vi "ME235ProjectVI.vi"() -> ()   [LabVIEW 2019]
uses:
  Serial - Settings.ctl
panel:
  out "XP2 Time":u8(graph)
  out "YP2 Time":u8(graph)
  out "YC1 Time":u8(graph)
  out "XC1 Time":u8(graph)
  in  "Speed Factor  Car 2":i32
  out "YC 1":u8[](array[numeric]) format="%x"
  out "XC1":u8[](array[numeric]) format="%x"
  out "YC2":u8[](array[numeric]) format="%x"
  out "XC2":u8[](array[numeric]) format="%x"
  in  "Set initial Y Car 2":dbl=1.3
  in  "Set initial X Car 2":dbl=2.6
  in  "?":bool
  in  "Time of Simulation in s":u8=5
  in  "command":u8=5
  out "XY Graph":cluster{u8[], u8[]}[](graph)
  out "Car Close By STOP":bool
  out "XY coordinates":u8[](array[numeric]) format="%x"
  out "return count":u32
  out "unsigned byte array":u8[](array[numeric])
  out "Packet Echo":u8[](array[numeric]) format="%x"
  out "read buffer":string
  in  "VISA resource name":refnum<visa-resource-name>="COM1"
  in  "Serial Settings":T1={"baud rate"=115200, "data bits"=8, "parity"=enum."None", "stop bits"=10, "flow control"=0} {"flow control" items=["None"=0, "XON/XOFF"=1, "RTS/CTS"=2, "DTR/DSR"=4]; "stop bits" items=["1.0"=10, "1.5"=15, "2.0"=20]; "data bits" min=5 max=8 step=1; "baud rate" items=["75"=75, "110"=110, "134"=134, "150"=150, "300"=300, "600"=600, "1200"=1200, "1800"=1800, "2400"=2400, "4800"=4800, "7200"=7200, "9600"=9600, "14400"=14400, "19200"=19200, "28800"=28800, "38400"=38400, "56000"=56000, "57600"=57600, "115200"=115200, "128000"=128000, "230400"=230400]}
  # "SIMULATION OF COLLISION DETECTION AND AVOIDANCE FOR 2 CARS"
  # "CAR 1 POSITION COMES FROM THE GPS INSIDE IT"
  # "CAR 1 INITIAL POS - X - 2, Y - 5, CAR 1 SPEED IS FACTOR 1"
  # "POSITIONS IN M, SPEED FACTOR"
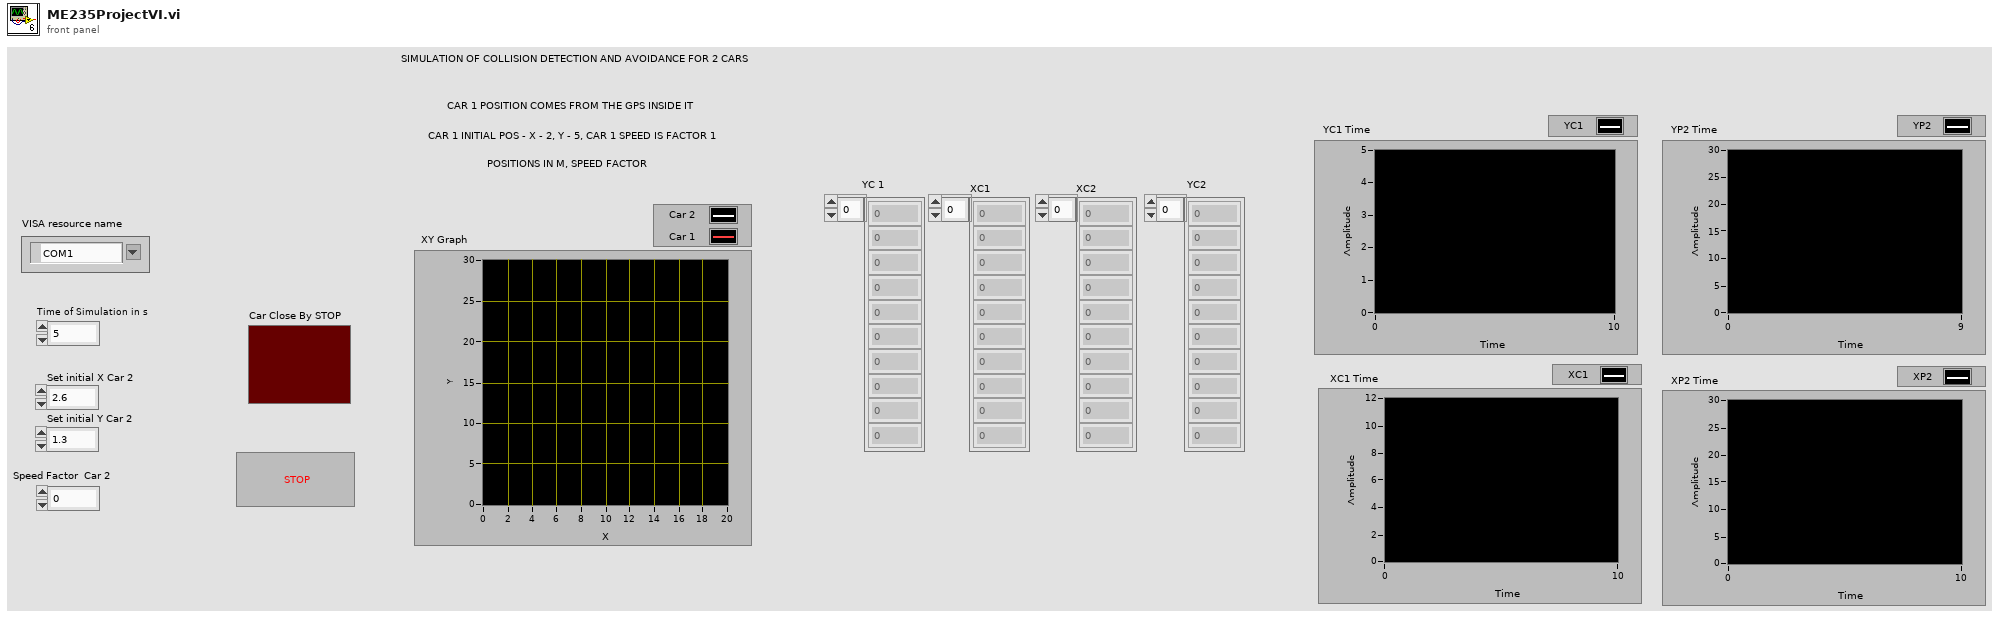
[diagram p1: front panel]
types:
  T1 = typedef "Serial - Settings.ctl" = cluster{"baud rate":u32, "data bits":u16, "parity":enum16{"None", "Odd", "Even", "Mark", "Space"}, "stop bits":u16, "flow control":u16}
  T2 = cluster{"Packet_Size":u8, "command":u8, "buffer":u8[]}
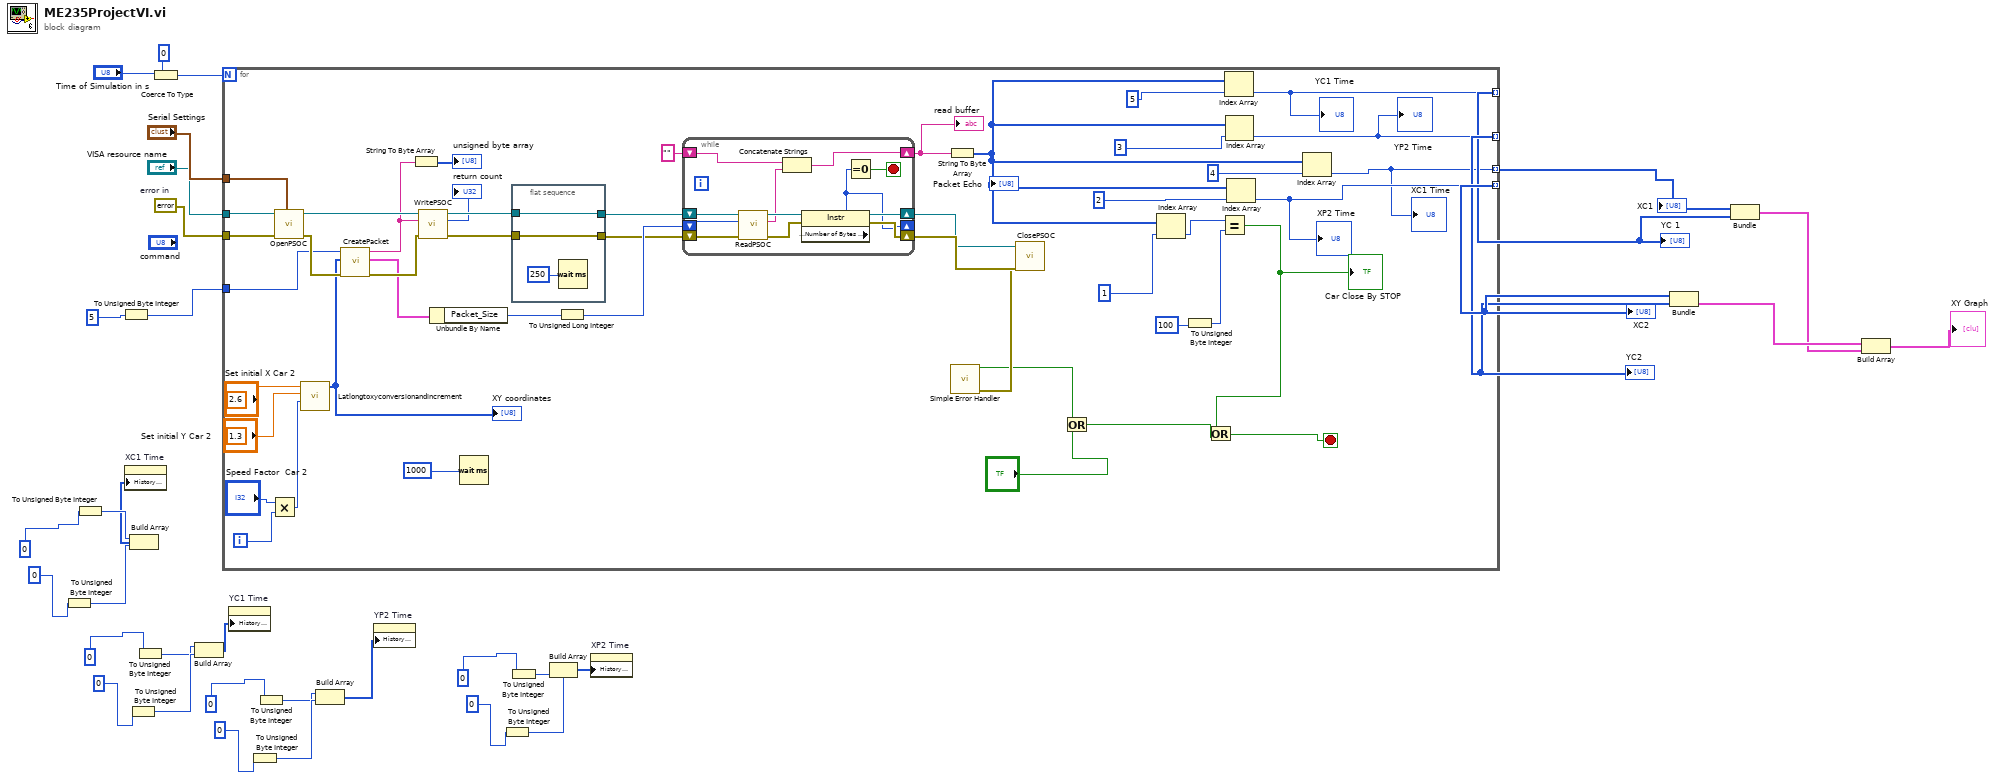
[diagram p0: block diagram]
diagram:
  w33 = errorcluster {"status"=FALSE, "code"=0, "source"=""}  # error in
  n1 = To Unsigned Byte Integer(number=0) -> (unsigned 8bit integer=w18:u8)
  n2 = To Unsigned Byte Integer(number=0) -> (unsigned 8bit integer=w17:u8)
  n3 = To Unsigned Byte Integer(number=5) -> (unsigned 8bit integer=w21:u8)
  n4 = To Unsigned Byte Integer(number=0) -> (unsigned 8bit integer=w13:u8)
  n5 = Build Array(w17, w18) -> (w16:u8[])
  n6 = property on="XC1 Time" class="WFChart (strict)"("History Data"=w16) -> ()  [unwired: 2 in, 2 out]
  n7 = To Unsigned Byte Integer(number=0) -> (unsigned 8bit integer=w12:u8)
  n8 = Coerce To Type(0:"Time of Simulation in s", 1:0) -> (2:w26:i32)
  n9 = Build Array(w12, w13) -> (w11:u8[])
  n10 = for {
    N: w26 -> [_]
    tunnel: "Serial Settings" -> [w82]
    tunnel: "VISA resource name" -> [w81]
    tunnel: w33 -> [w80]
    tunnel: w21 -> [w67]
    tunnel: [w37] -> w32 mode=indexing
    tunnel: [w38] -> w31 mode=indexing
    tunnel: [w36] -> w25 mode=indexing
    tunnel: [w39] -> w24 mode=indexing
    i -> [w44]
    stop <- w40 stop-if-true
    n11 = Multiply(x="Speed Factor  Car 2", y=w44) -> (x*y=w43:i32)
    n12 = call "OpenPSOC.vi"("Serial Settings"=w82, "error in"=w80, "VISA resource name"=w81) -> ("error out"=w79:errorcluster, "VISA resource name out"=w77:refnum<visa-resource-name>)  [unwired: 7 in]
    n13 = call "Latlongtoxyconversionandincrement.vi"("Numeric 2"=w43, "Numeric 3"=1.3, "Numeric"=2.6) -> ("Array"=w59:u8[])  [unwired: 8 in]
    "XY coordinates" <- w59
    n14 = call "CreatePacket.vi"("error in"=w79, "data"=w59, "command"=w67) -> ("error out"=w78:errorcluster, "output cluster"=w73:T2, "Command String"=w66:string)  [unwired: 6 in]
    n15 = String To Byte Array(string=w66) -> (unsigned byte array=→"unsigned byte array":u8[])
    n16 = call "WritePSOC.vi"("error in"=w78, "write buffer"=w66, "VISA resource name"=w77) -> ("error out"=w70:errorcluster, "return count"=→"return count":u32, "VISA resource name out"=w76:refnum<visa-resource-name>)  [unwired: 5 in]
    n17 = Unbundle By Name(w73) -> ("Packet_Size"=w72:u8)
    n18 = Wait (ms)(milliseconds to wait=u32 1000) -> ()  [unwired: 1 out]
    n19 = flat-sequence {
      tunnel: w76 -> [w97]
      tunnel: [w97] -> w74
      tunnel: [w95] -> w69
      tunnel: w70 -> [w95]
      frame #0 {
        n20 = Wait (ms)(milliseconds to wait=u32 250) -> ()  [unwired: 1 out]
      }
    }
    n21 = To Unsigned Long Integer(number=w72) -> (unsigned 32bit integer=w71:u32)
    n22 = while {
      shift-right: [w90] -> w63
      shift-left: w74 -> [w94]
      shift-right: [w88] -> w75
      shift-left: w69 -> [w92]
      shift-right: [w85] -> w62
      shift-left: "" -> [w84]
      shift-right: [w83] -> _
      shift-left: w71 -> [w93]
      stop <- w87 stop-if-true
      n23 = call "ReadPSOC.vi"("error in"=w92, "byte count"=w93, "VISA resource name"=w94) -> ("error out"=w89:errorcluster, "read buffer"=w86:string, "VISA resource name out"=w91:refnum<visa-resource-name>)  [unwired: 5 in]
      n24 = Concatenate Strings(w84, w86) -> (w85:string)
      n25 = property class="Instr"(reference=w91, error in=w89) -> (reference out=w90:refnum<visa-resource-name>, error out=w88:errorcluster, "Serial Settings:Number of Bytes at Serial Port"=w83:u32)
      n26 = Equal To 0?(x=w83) -> (x = 0?=w87:bool)
    }
    "read buffer" <- w62
    n27 = String To Byte Array(string=w62) -> (unsigned byte array=w46:u8[])
    "Packet Echo" <- w46
    n28 = call "ClosePSOC.vi"("error in"=w75, "VISA resource name"=w63) -> ("error out"=w68:errorcluster)  [unwired: 9 in]
    n29 = call <vilib>:"Simple Error Handler.vi"("error in (no error)"=w68) -> ("error?"=w54:bool)  [unwired: 4 in, 4 out]
    n30 = Or(x="?", y=w54) -> (x .or. y?=w41:bool)
    n31 = Index Array(array=w46, index=1) -> (element=w57:u8)
    n32 = To Unsigned Byte Integer(number=100) -> (unsigned 8bit integer=w55:u8)
    n33 = Equal?(x=w57, y=w55) -> (x = y?=w42:bool)
    "Car Close By STOP" <- w42
    n34 = Or(x=w42, y=w41) -> (x .or. y?=w40:bool)
    n35 = Index Array(array=w46, index=5) -> (element=w39:u8)
    "YC1 Time" <- w39
    n36 = Index Array(array=w46, index=3) -> (element=w38:u8)
    "YP2 Time" <- w38
    n37 = Index Array(array=w46, index=2) -> (element=w37:u8)
    "XP2 Time" <- w37
    n38 = Index Array(array=w46, index=4) -> (element=w36:u8)
    "XC1 Time" <- w36
  }
  "XC2" <- w32
  "YC2" <- w31
  "XC1" <- w25
  "YC 1" <- w24
  n39 = property on="YC1 Time" class="WFChart (strict)"("History Data"=w11) -> ()  [unwired: 2 in, 2 out]
  n40 = To Unsigned Byte Integer(number=0) -> (unsigned 8bit integer=w8:u8)
  n41 = To Unsigned Byte Integer(number=0) -> (unsigned 8bit integer=w7:u8)
  n42 = Build Array(w7, w8) -> (w6:u8[])
  n43 = property on="YP2 Time" class="WFChart (strict)"("History Data"=w6) -> ()  [unwired: 2 in, 2 out]
  n44 = To Unsigned Byte Integer(number=0) -> (unsigned 8bit integer=w3:u8)
  n45 = To Unsigned Byte Integer(number=0) -> (unsigned 8bit integer=w2:u8)
  n46 = Build Array(w2, w3) -> (w1:u8[])
  n47 = property on="XP2 Time" class="WFChart (strict)"("History Data"=w1) -> ()  [unwired: 2 in, 2 out]
  n48 = Bundle(w32, w31) -> (w30:cluster{u8[], u8[]})  [unwired: 1 in]
  n49 = Bundle(w25, w24) -> (w23:cluster{u8[], u8[]})  [unwired: 1 in]
  n50 = Build Array(w30, w23) -> (→"XY Graph":cluster{u8[], u8[]}[])
